vi "ParseSWI.vi"(8 "error in (no error)":errorcluster, 9 "Master Device in":refnum<class "Master Device.lvclass">, 10 "Current Variables":T1[](array[typedef]), 11 "Novatech in":refnum<class "Novatech.lvclass">) -> (0 "error out":errorcluster, 2 "Master Device out":refnum<class "Master Device.lvclass">, 3 "Novatech out":refnum<class "Novatech.lvclass">)   [LabVIEW 2013, in "Novatech.lvclass"]
doc: "All specific devices will override ParseSWI method (i.e. you can delete the parent call)\n (1) Get devices data from private data\n (2) Get Slave Info (Ramp List) from Master Device\n (3) Parse data into \"prepared HWI\" which is in reverse order to match Ramp List."
uses:
  Novatech.lvclass
  Device/Device.lvclass
  TypeDefs/Active procedure variables.ctl
  Master Device/Master Device.lvclass
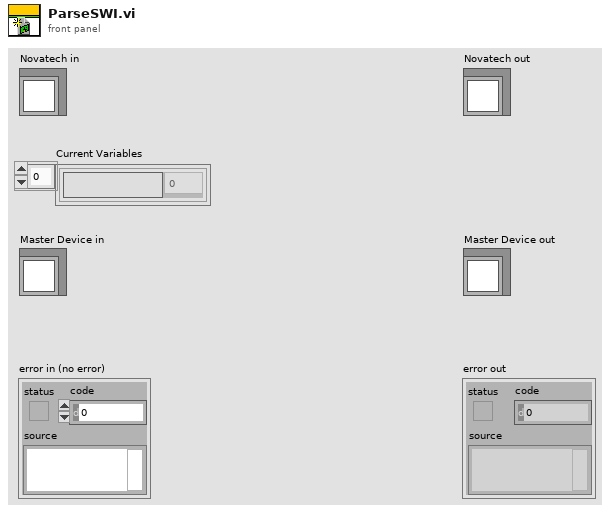
[diagram p1: front panel]
types:
  T1 = typedef "Active procedure variables.ctl" = cluster{"Procedure variable":string, "Value":dbl}
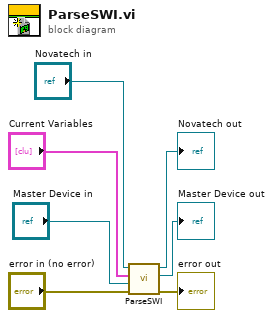
[diagram p0: block diagram]
diagram:
  n1 = call-parent "ParseSWI.vi"("error in (no error)"="error in (no error)", "Master Device in"="Master Device in", "Current Variables"="Current Variables", "Device in"="Novatech in") -> ("error out"=→"error out":errorcluster, "Master Device out"=→"Master Device out":refnum<class "Master Device.lvclass">, "Device out"=→"Novatech out":refnum<class "Novatech.lvclass">)  [unwired: 5 in]
